vi "Import Private Key.vi"(7 "Crypto Provider":T1, 8 "error in (no error)":errorcluster, 11 "PrivateKeyBlob":u8[](array[numeric])) -> (0 "error out":errorcluster, 3 "Imported CngKey out":refnum<k24>)   [LabVIEW 2021, in "dotNET Crypto Key Management.lvlib"]
uses:
  CNG Provider Type.ctl
  System.Core
  dotNET Crypto Key Management.lvlib
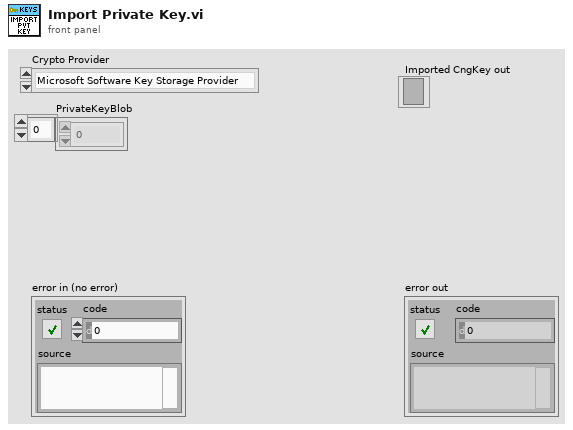
[diagram p1: front panel]
types:
  T1 = typedef "dotNET Crypto Key Management.lvlib/CNG Provider Type.ctl" = enum16{"Microsoft Software Key Storage Provider", "Microsoft Platform Crypto Provider"}
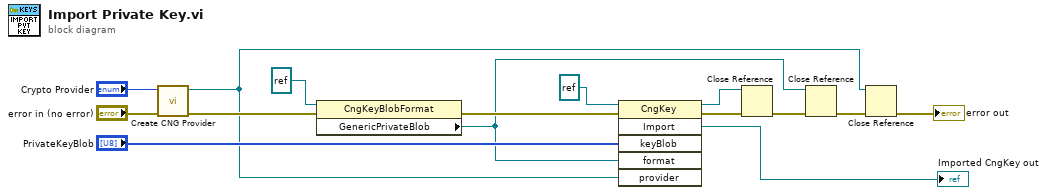
[diagram p0: block diagram]
diagram:
  n1 = call "Create CNG Provider.vi"("error in (no error)"="error in (no error)", "Crypto Provider"="Crypto Provider") -> ("error out"=w12:errorcluster, "CngProvider"=w4:refnum<k24>)  [unwired: 8 in]
  n2 = property class="CngKeyBlobFormat"(reference=refnum<k24> refnum ("format"), error in=w12) -> (error out=w13:errorcluster, "GenericPrivateBlob"=w6:refnum<k24>)  [unwired: 1 out]
  n3 = invoke class="CngKey" method="Import"(reference=refnum<k24> refnum, error in=w13, "keyBlob"="PrivateKeyBlob", "format"=w6, "provider"=w4) -> (reference out=w8:refnum<k24>, error out=w9:errorcluster, "Import"=→"Imported CngKey out":refnum<k24>)  [unwired: 1 in, 3 out]
  n4 = Close Reference(reference=w8, error in (no error)=w9) -> (error out=w7:errorcluster)
  n5 = Close Reference(reference=w6, error in (no error)=w7) -> (error out=w5:errorcluster)
  n6 = Close Reference(reference=w4, error in (no error)=w5) -> (error out=→"error out":errorcluster)
